vi "Open Process Data TypeDef.vi"(8 "error in (no error)":errorcluster, 10 "Panel Bounds":T1, 11 "Path to Library":path) -> (0 "error out":errorcluster, 3 "ProcessData Ref":refnum<vi>)   [LabVIEW 2020]
uses:
  <vilib>/Utility/miscctls.llb/LVRectTypeDef.ctl
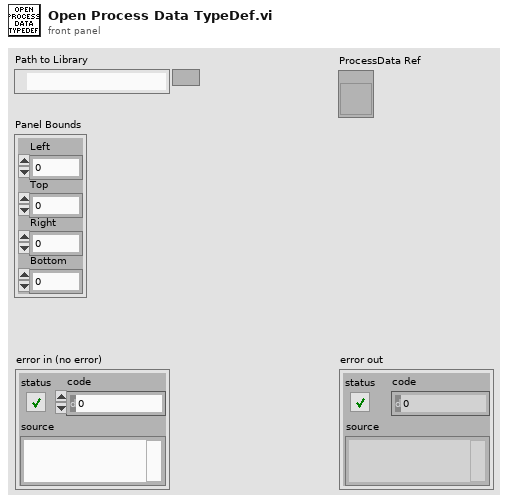
[diagram p1: front panel]
types:
  T1 = typedef "LVRectTypeDef.ctl" = cluster{"Left":i16, "Top":i16, "Right":i16, "Bottom":i16}
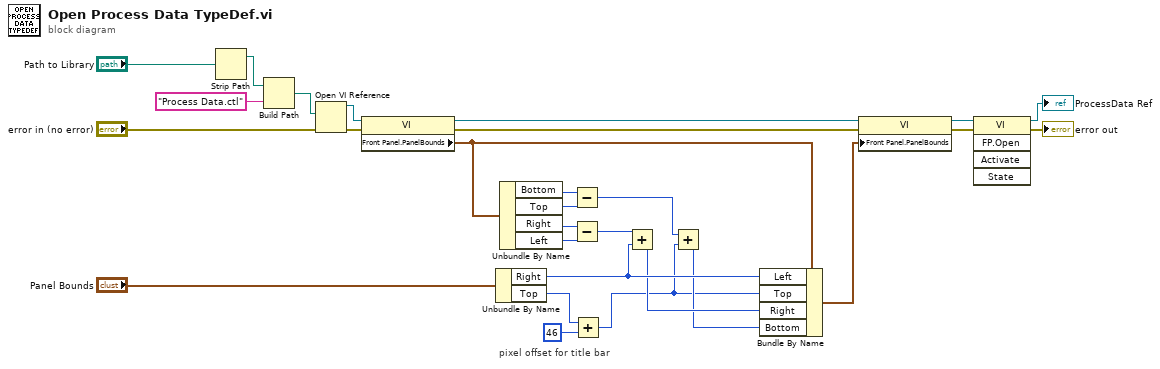
[diagram p0: block diagram]
diagram:
  # "pixel offset for title bar"
  n1 = Strip Path(path="Path to Library") -> (stripped path=w28:path)  [unwired: 1 out]
  n2 = Build Path(base path=w28, name or relative path="Process Data.ctl") -> (appended path=w26:path)
  n3 = Open VI Reference(vi path=w26, error in (no error)="error in (no error)") -> (vi reference=w21:refnum<vi>, error out=w18:errorcluster)  [unwired: 4 in]
  n4 = property class="VI"(reference=w21, error in=w18) -> (reference out=w20:refnum<vi>, error out=w17:errorcluster, "Front Panel.PanelBounds"=w10:T1)
  n5 = Unbundle By Name("Panel Bounds") -> ("Right"=w7:i16, "Top"=w3:i16)
  n6 = Unbundle By Name(w10) -> ("Bottom"=w11:i16, "Top"=w14:i16, "Right"=w13:i16, "Left"=w12:i16)
  n7 = Subtract(x=w11, y=w14) -> (x-y=w5:i16)
  n8 = Subtract(x=w13, y=w12) -> (x-y=w8:i16)
  n9 = Add(x=w3, y=i16 46) -> (x+y=w1:i16)
  n10 = Add(x=w8, y=w7) -> (x+y=w6:i16)
  n11 = Add(x=w5, y=w1) -> (x+y=w4:i16)
  n12 = Bundle By Name(cluster=w10, "Left"=w7, "Top"=w1, "Right"=w6, "Bottom"=w4) -> (w9:T1)
  n13 = property class="VI"(reference=w20, error in=w17, "Front Panel.PanelBounds"=w9) -> (reference out=w16:refnum<vi>, error out=w19:errorcluster)
  n14 = invoke class="VI" method="FP.Open"(reference=w16, error in=w19) -> (reference out=→"ProcessData Ref":refnum<vi>, error out=→"error out":errorcluster)  [unwired: 3 in, 3 out]
